vi "ACQ stop and clear.vi"(8 "error in (no error)":errorcluster, 11 "Tasks ref in":T1) -> (0 "error out":errorcluster)   [LabVIEW 2014]
uses:
  Kontrolki/KartaDAQ/ACQ all read tasks.ctl
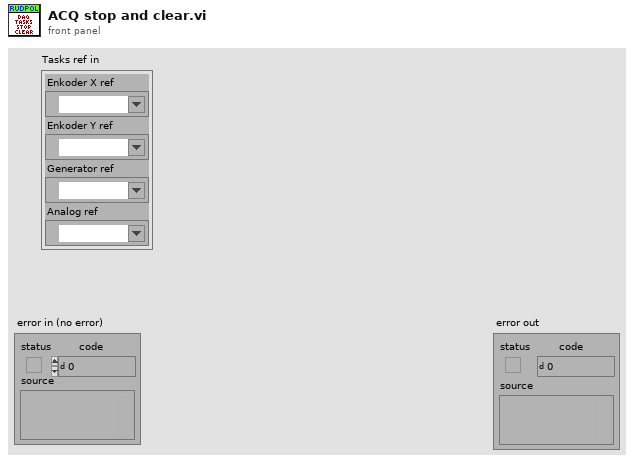
[diagram p1: front panel]
types:
  T1 = typedef "ACQ all read tasks.ctl" = cluster{"Enkoder X ref":refnum<k21>, "Enkoder Y ref":refnum<k21>, "Generator ref":refnum<k21>, "Analog ref":refnum<k21>}
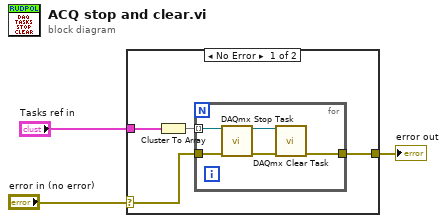
[diagram p0: block diagram]
diagram:
  n1 = case shown="No Error" "error in (no error)" {
    selector: "error in (no error)" -> [w5 w13]
    tunnel: [w4 w13] -> w2
    tunnel: "Tasks ref in" -> [w6 _]
    frame No Error {
      n2 = Cluster To Array(cluster=w6) -> (array=w7:refnum<k21>[])
      n3 = for {
        tunnel: w7 -> [w12] mode=indexing
        tunnel: w5 -> [w11]
        tunnel: [w8] -> w4
        n4 = call <vilib>:"DAQmx Stop Task.vi"("task/channels in"=w12, "error in"=w11) -> ("task out"=w9:refnum<k21>, "error out"=w10:errorcluster)  [unwired: 12 in]
        n5 = call <vilib>:"DAQmx Clear Task.vi"("task in"=w9, "error in"=w10) -> ("error out"=w8:errorcluster)  [unwired: 13 in]
      }
    }
    frame Error {
    }
  }
  "error out" <- w2
